vi "Number of Rows.vi"(8 "error in (no error)":errorcluster, 11 "PQ Result in":refnum<class "PQ Result.lvclass">) -> (0 "error out":errorcluster, 2 "Number of Rows":i32, 3 "PQ Result out":refnum<class "PQ Result.lvclass">)   [LabVIEW 2016, in "PQ Result.lvclass"]
uses:
  PQ Result.lvclass
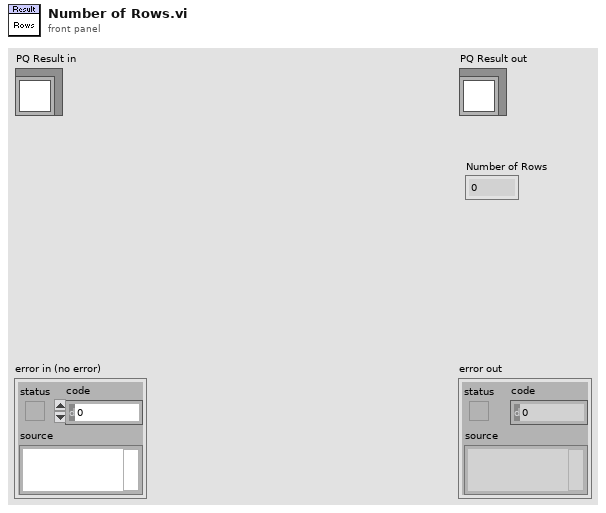
[diagram p1: front panel]
types:
  T1 = typedef "PQ Result.lvclass/Result Status.ctl" = enum32{"PGRES_EMPTY_QUERY", "PGRES_COMMAND_OK", "PGRES_TUPLES_OK", "PGRES_COPY_OUT", "PGRES_COPY_IN", "PGRES_BAD_RESPONSE", "PGRES_NONFATAL_ERROR", "PGRES_FATAL_ERROR", "PGRES_COPY_BOTH", "PGRES_SINGLE_TUPLE"}
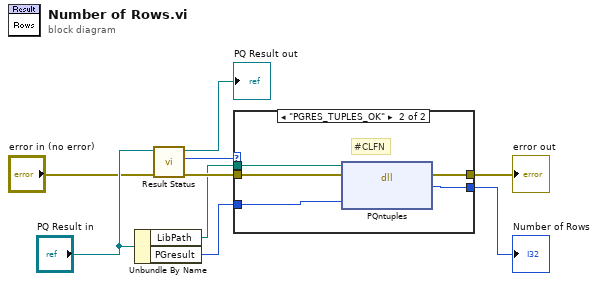
[diagram p0: block diagram]
diagram:
  n1 = Unbundle By Name("PQ Result in") -> ("LibPath"=w1:path, "PGresult"=w5:u32)
  n2 = call "Result Status.vi"("error in (no error)"="error in (no error)", "PQ Result in"="PQ Result in") -> ("error out"=w2:errorcluster, "Result Status"=w4:T1, "PQ Result out"=→"PQ Result out":refnum<class "PQ Result.lvclass">)  [unwired: 7 in]
  n3 = case shown="\"PGRES_TUPLES_OK\"" w4 {
    tunnel: [w10 w15] -> w9
    tunnel: [_ w14] -> w8
    tunnel: w2 -> [w10 w13]
    tunnel: w5 -> [_ w12]
    tunnel: w1 -> [_ w11]
    frame "PGRES_EMPTY_QUERY", Default {
    }
    frame "PGRES_TUPLES_OK" {
      # "#CLFN"
      n4 = dll-call lib="libpq.*" fn="PQntuples"(path in=w11, error in=w13, "PGresult"=w12) -> (error out=w15:errorcluster, "PQntuples"=w14:i32)  [unwired: 2 in, 1 out]
    }
  }
  "error out" <- w9
  "Number of Rows" <- w8
